vi "Read States.vi"(8 "error in (no error)":errorcluster, 11 "Vessel in":refnum<class "Vessel.lvclass">) -> (0 "error out":errorcluster, 2 "States":T1, 3 "Vessel out":refnum<class "Vessel.lvclass">)   [LabVIEW 2014, in "Vessel.lvclass"]
uses:
  Vessel.lvclass
  Vessel.lvclass/Vessel.ctl
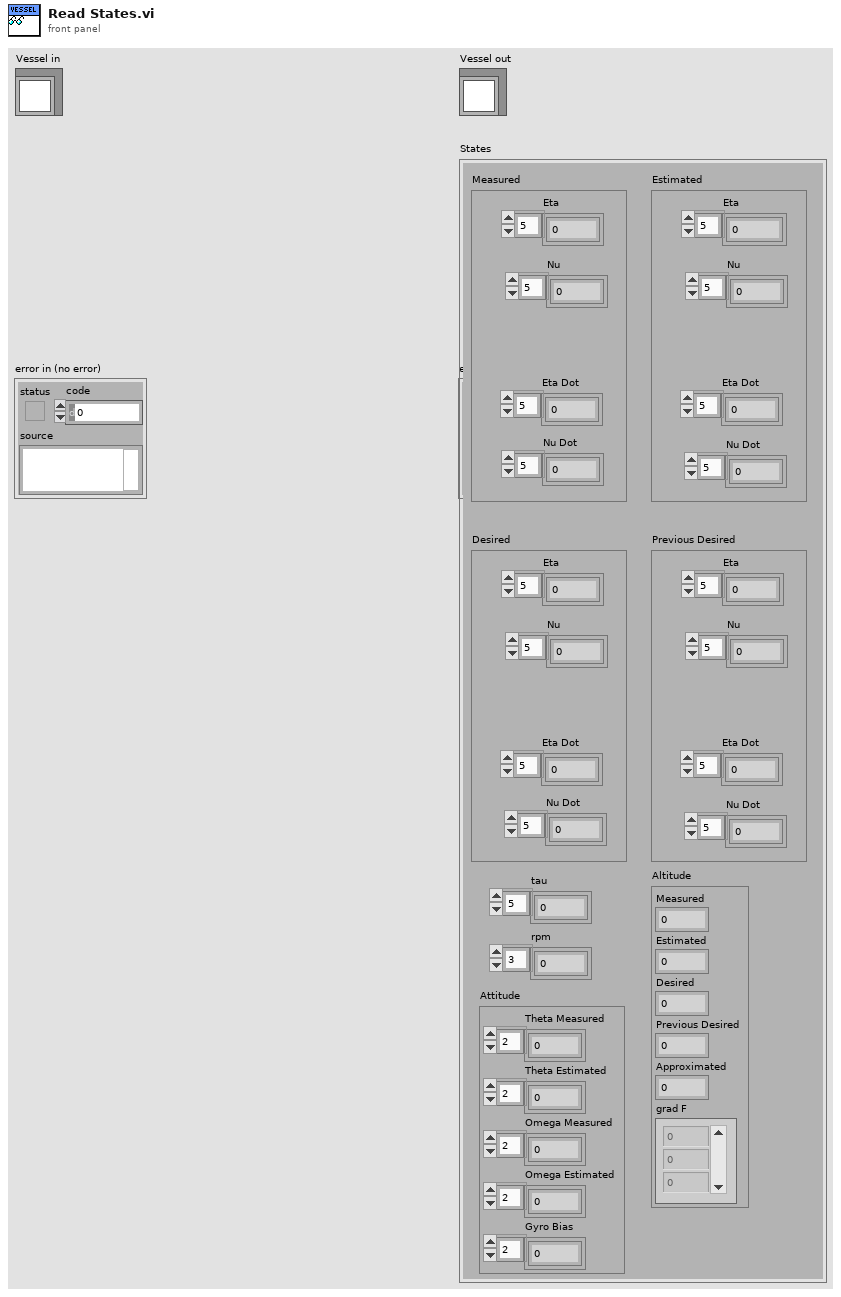
[diagram p1: front panel]
types:
  T1 = cluster{"Measured":cluster{"Eta":dbl[], "Nu":dbl[], "Eta Dot":dbl[], "Nu Dot":dbl[]}, "Estimated":cluster{"Eta":dbl[], "Nu":dbl[], "Eta Dot":dbl[], "Nu Dot":dbl[]}, "Desired":cluster{"Eta":dbl[], "Nu":dbl[], "Eta Dot":dbl[], "Nu Dot":dbl[]}, "Previous Desired":cluster{"Eta":dbl[], "Nu":dbl[], "Eta Dot":dbl[], "Nu Dot":dbl[]}, "tau":dbl[], "Altitude":cluster{"Measured":dbl, "Estimated":dbl, "Desired":dbl, "Previous Desired":dbl, "Approximated":dbl, "grad F":dbl[]}, "rpm":dbl[], "Attitude":cluster{"Theta Measured":dbl[], "Theta Estimated":dbl[], "Omega Measured":dbl[], "Omega Estimated":dbl[], "Gyro Bias":dbl[]}}
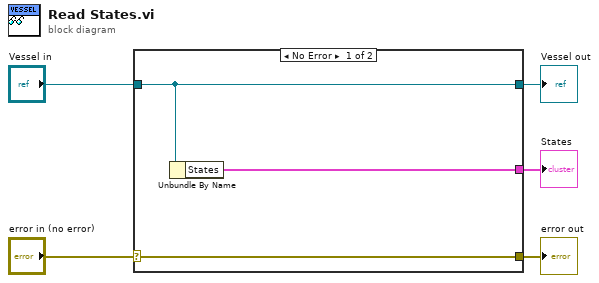
[diagram p0: block diagram]
diagram:
  n1 = case shown="No Error" "error in (no error)" {
    selector: "error in (no error)" -> [w8 w9]
    tunnel: [w8 w9] -> w4
    tunnel: [w7 w10] -> w2
    tunnel: "Vessel in" -> [w7 w10]
    tunnel: [w6 _] -> w1
    frame No Error {
      n2 = Unbundle By Name(w7) -> ("States"=w6:T1)
    }
    frame Error {
    }
  }
  "error out" <- w4
  "Vessel out" <- w2
  "States" <- w1
